vi "ex1_4b.vi"() -> ()   [LabVIEW 2017]
panel:
  out "filtered and raw data":dynamicdata(graph)
  out "Identified high frequency":u16
  out "Identified  low frequency":u16
  in  "stop":bool
  out "Waveform Graph 2":dynamicdata(graph)
  out "Waveform Graph":dynamicdata(graph)
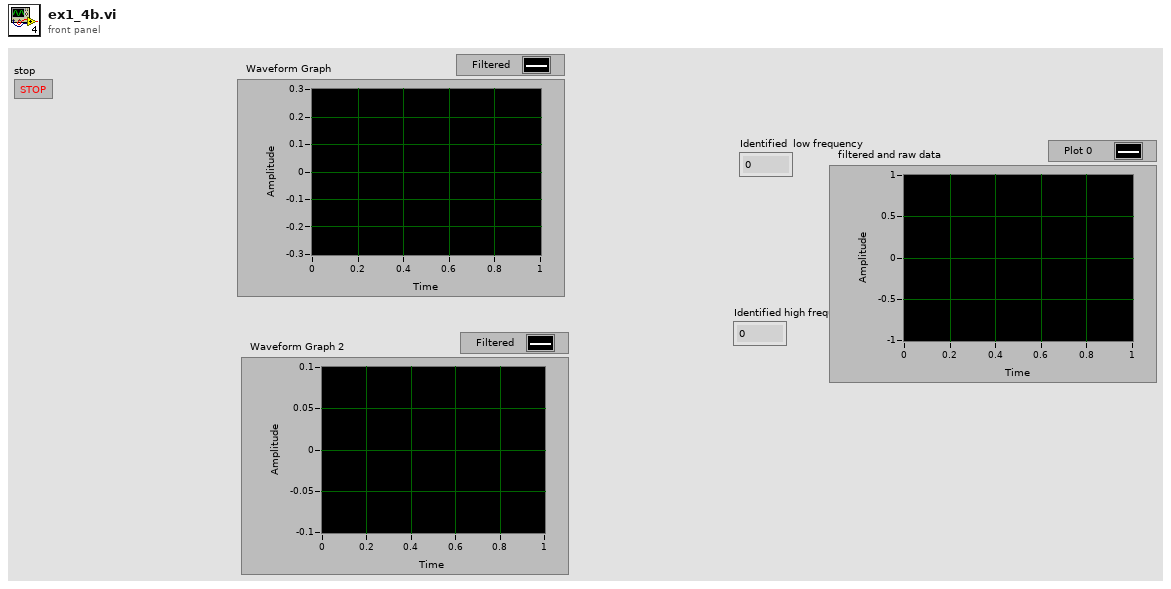
[diagram p1: front panel]
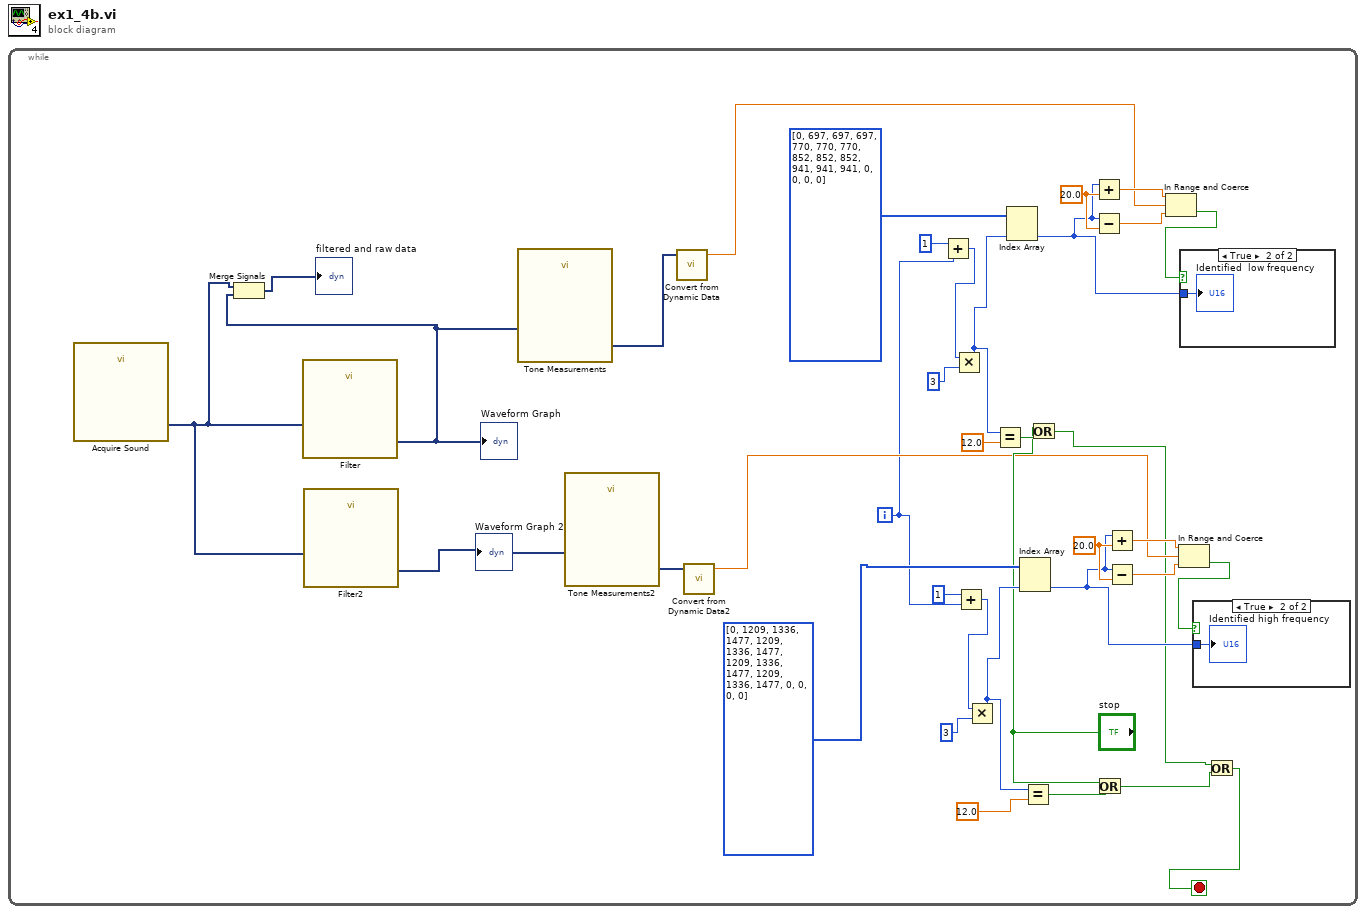
[diagram p0: block diagram]
diagram:
  n1 = while {
    i -> [w8]
    stop <- w4 stop-if-true
    w18 = 20.0 ("y")
    w29 = 20.0 ("y")
    n2 = call "Acquire Sound"() -> ("Data"=w2:dynamicdata)  [unwired: 18 in, 1 out]
    n3 = call "Filter"("Signal"=w2) -> ("Filtered Signal"=w1:dynamicdata)  [unwired: 9 in, 1 out]
    "Waveform Graph" <- w1
    n4 = Merge Signals(w2, w1) -> (→"filtered and raw data":dynamicdata)
    n5 = call "Filter2"("Signal"=w2) -> ("Filtered Signal"=w37:dynamicdata)  [unwired: 9 in, 1 out]
    "Waveform Graph 2" <- w37
    n6 = call "Tone Measurements"("Signals"=w1) -> ("Frequency"=w26:dynamicdata)  [unwired: 9 in, 1 out]
    n7 = call "Tone Measurements2"("Signals"=w37) -> ("Frequency"=w10:dynamicdata)  [unwired: 9 in, 1 out]
    n8 = call "Convert from Dynamic Data"("Dynamic Data Type"=w26) -> ("Scalar"=w25:dbl)  [unwired: 3 in]
    n9 = call "Convert from Dynamic Data2"("Dynamic Data Type"=w10) -> ("Scalar"=w9:dbl)  [unwired: 3 in]
    n10 = Add(x=1, y=w8) -> (x+y=w30:i32)
    n11 = Multiply(x=w30, y=3) -> (x*y=w33:i32)
    n12 = Add(x=1, y=w8) -> (x+y=w19:i32)
    n13 = Multiply(x=w19, y=3) -> (x*y=w22:i32)
    n14 = Equal?(x=w33, y=12.0) -> (x = y?=w32:bool)
    n15 = Index Array(array=u16[] [0, 697, 697, 697, 770, 770, 770, 852, 852, 852, 941, 941, 941, 0, 0, 0, 0], index #2=w33) -> (element #2=w7:u16)  [unwired: 1 in, 1 out]
    n16 = Index Array(array=u16[] [0, 1209, 1336, 1477, 1209, 1336, 1477, 1209, 1336, 1477, 1209, 1336, 1477, 0, 0, 0, 0], index #2=w22) -> (element #2=w14:u16)  [unwired: 1 in, 1 out]
    n17 = Equal?(x=w22, y=12.0) -> (x = y?=w21:bool)
    n18 = Or(x="stop", y=w32) -> (x .or. y?=w5:bool)
    n19 = Add(x=w7, y=w29) -> (x+y=w28:dbl)
    n20 = Subtract(x=w7, y=w29) -> (x-y=w27:dbl)
    n21 = Or(x="stop", y=w21) -> (x .or. y?=w6:bool)
    n22 = Add(x=w14, y=w18) -> (x+y=w17:dbl)
    n23 = Subtract(x=w14, y=w18) -> (x-y=w16:dbl)
    n24 = In Range and Coerce(upper limit=w28, x=w25, lower limit=w27) -> (In Range?=w24:bool)  [unwired: 1 out]
    n25 = In Range and Coerce(upper limit=w17, x=w9, lower limit=w16) -> (In Range?=w15:bool)  [unwired: 1 out]
    n26 = case shown="True" w24 {
      tunnel: w7 -> [_ w39]
      frame False {
      }
      frame True {
        "Identified  low frequency" <- w39
      }
    }
    n27 = case shown="True" w15 {
      tunnel: w14 -> [_ w38]
      frame False {
      }
      frame True {
        "Identified high frequency" <- w38
      }
    }
    n28 = Or(x=w5, y=w6) -> (x .or. y?=w4:bool)
  }
